vi "SubPanelAdd.vi"(0 "Add in":refnum<class "Add.lvclass">, 1 "B":dbl, 5 "A":dbl, 7 "user event out":refnum<user-event>, 9 "event source":refnum<user-event>, 11 "error in (no error)":errorcluster, 12 "Calculate":bool) -> (4 "Add out":refnum<class "Add.lvclass">, 6 "C":dbl, 15 "error out":errorcluster)   [LabVIEW 2023, in "Add.lvclass"]
uses:
  Add.lvclass
  Arithmetic/Arithmetic.lvclass
  Add.lvclass/Add.ctl
panel:
  # "ADDITION"
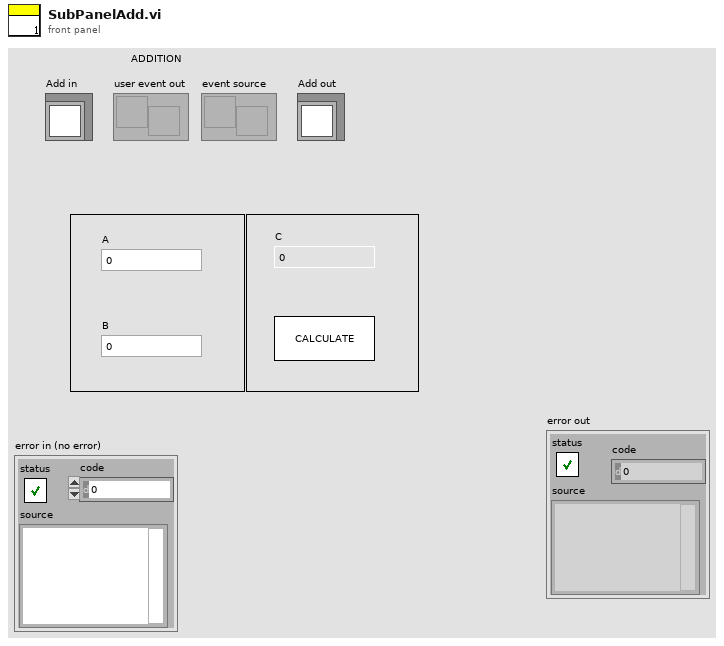
[diagram p1: front panel]
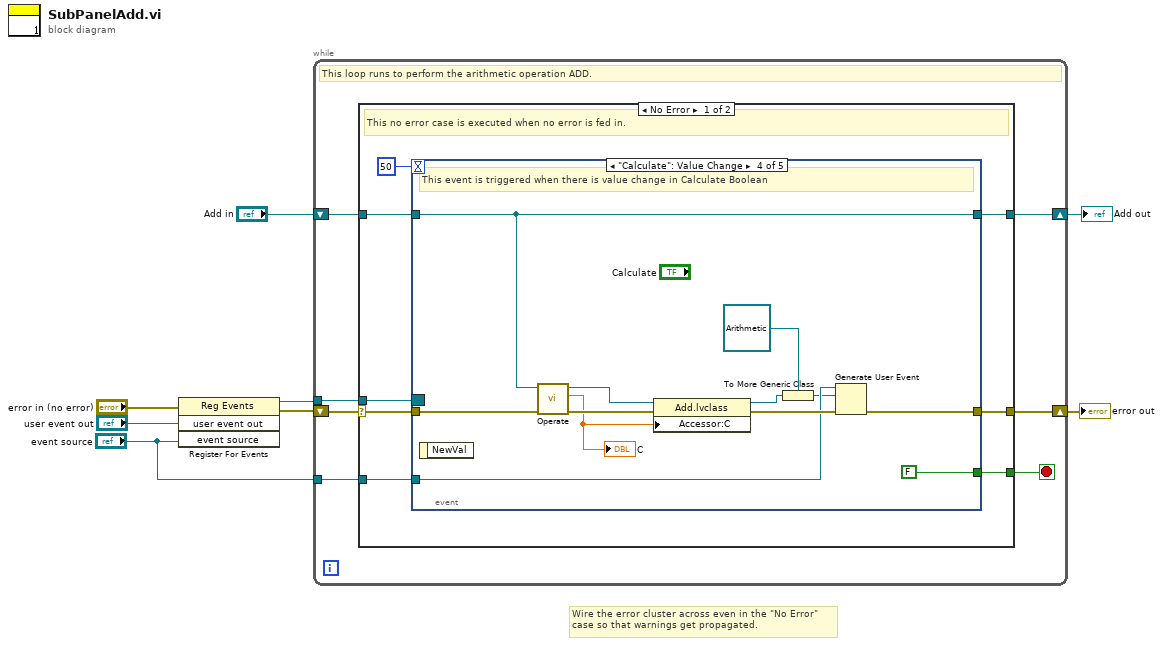
[diagram p0: block diagram]
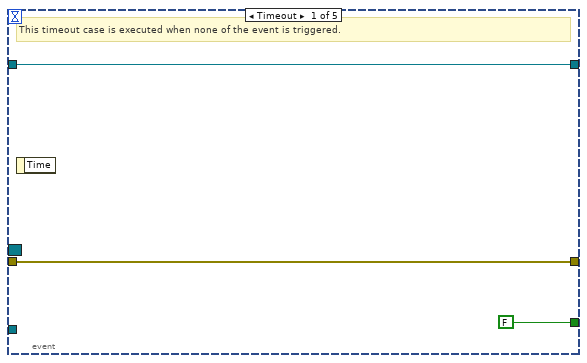
[diagram p2: hidden frame]
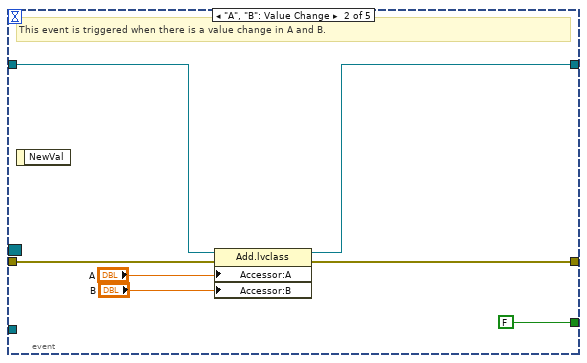
[diagram p3: hidden frame]
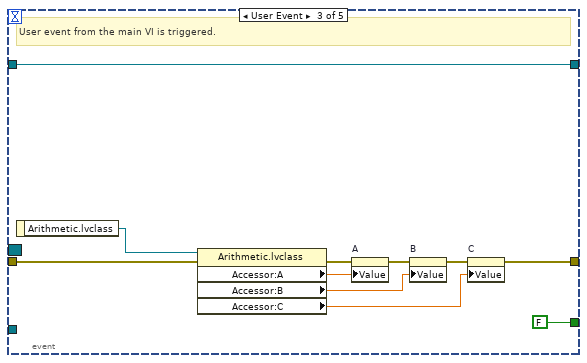
[diagram p4: hidden frame]
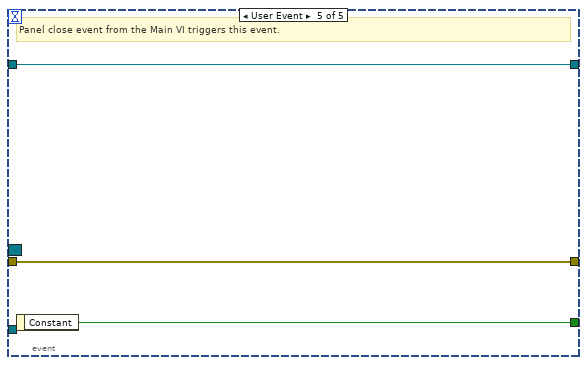
[diagram p5: hidden frame]
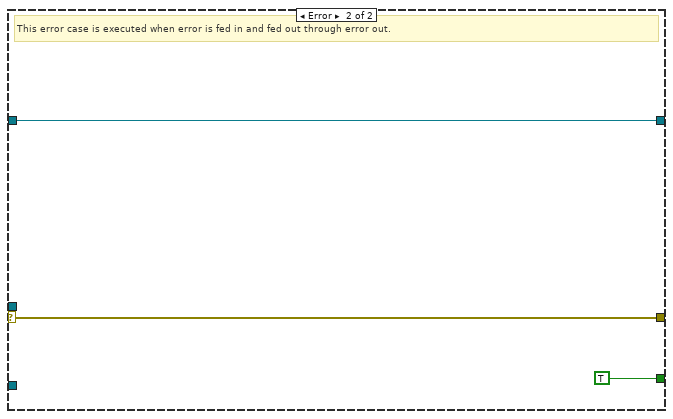
[diagram p6: hidden frame]
diagram:
  # "Wire the error cluster across even in the \"No Error\"\ncase so that warnings get propagated."
  n1 = register-events(error in="error in (no error)", "user event out", "event source") -> (reference out=w1:refnum<event-registration>, error out=w6:errorcluster)  [unwired: 1 in]
  n2 = while {
    shift-right: [w14] -> w4
    shift-left: w6 -> [w15]
    shift-right: [w12] -> w7
    shift-left: "Add in" -> [w13]
    tunnel: w1 -> [w11]
    tunnel: "event source" -> [w9]
    stop <- w10 stop-if-true
    # "This loop runs to perform the arithmetic operation ADD."
    n3 = case shown="No Error" w15 {
      selector: w15 -> [w23 w62]
      tunnel: [w22 w62] -> w14
      tunnel: [w20 w61] -> w12
      tunnel: w13 -> [w21 w61]
      tunnel: w11 -> [w18 _]
      tunnel: [w17 TRUE] -> w10
      tunnel: w9 -> [w16 _]
      frame No Error {
        # "This no error case is executed when no error is fed in."
        n4 = event shown="[3] \"Calculate\": Value Change" {
          selector: w18 -> [_ _ _ _ _]
          dyn-events: _ -> [_ _ _ _ _]
          timeout: 50 -> [_ _ _ _ _]
          tunnel: w23 -> [w26 w33 w44 w56 w59]
          tunnel: [w26 w32 w43 w53 w59] -> w22
          tunnel: w21 -> [w25 w28 w41 w47 w58]
          tunnel: [w25 w27 w41 w47 w58] -> w20
          tunnel: [FALSE FALSE FALSE ("Constant") FALSE w57] -> w17
          tunnel: w16 -> [_ _ _ w48 _]
          event Timeout {
            # "This timeout case is executed when none of the event is triggered."
            n5 = event-data() -> ()  [unwired: 1 in, 1 out]
          }
          event "A", "B": Value Change {
            # "This event is triggered when there is a value change in A and B."
            n6 = event-data() -> ()  [unwired: 1 in, 1 out]
            n7 = property class="Add.lvclass"(reference=w28, error in=w33, "Accessor:A"="A", "Accessor:B"="B") -> (reference out=w27:refnum<class "Add.lvclass">, error out=w32:errorcluster)
          }
          event User Event {
            # "User event from the main VI is triggered."
            n8 = event-data() -> ("Arithmetic.lvclass"=w34:refnum<class "Arithmetic.lvclass">)  [unwired: 1 in]
            n9 = property class="Arithmetic.lvclass"(reference=w34, error in=w44) -> (error out=w40:errorcluster, "Accessor:A"=w39:dbl, "Accessor:B"=w36:dbl, "Accessor:C"=w35:dbl)  [unwired: 1 out]
            n10 = property on="A" class="DigNum (strict)"(error in=w40, "Value"=w39) -> (error out=w38:errorcluster)  [unwired: 1 in, 1 out]
            n11 = property on="B" class="DigNum (strict)"(error in=w38, "Value"=w36) -> (error out=w37:errorcluster)  [unwired: 1 in, 1 out]
            n12 = property on="C" class="DigNum (strict)"(error in=w37, "Value"=w35) -> (error out=w43:errorcluster)  [unwired: 1 in, 1 out]
          }
          event "Calculate": Value Change {
            # "This event is triggered when there is value change in Calculate Boolean"
            n13 = event-data() -> ()  [unwired: 1 in, 1 out]
            n14 = call-dynamic "Operate.vi"("error in (no error)"=w56, "Add in"=w47) -> ("error out"=w54:errorcluster, "C"=w50:dbl, "Add out"=w51:refnum<class "Add.lvclass">)  [unwired: 7 in]
            "C" <- w50
            n15 = property class="Add.lvclass"(reference=w51, error in=w54, "Accessor:C"=w50) -> (reference out=w49:refnum<class "Add.lvclass">, error out=w52:errorcluster)
            n16 = To More Generic Class(target class=refnum<class "Arithmetic.lvclass"> refnum ("Arithmetic.lvclass"), reference=w49) -> (generic class reference=w46:refnum<class "Arithmetic.lvclass">)
            n17 = Generate User Event(user event=w48, event data cluster=w46, error in=w52) -> (error out=w53:errorcluster)  [unwired: 1 in, 1 out]
          }
          event User Event {
            # "Panel close event from the Main VI triggers this event."
            n18 = event-data() -> ("Constant"=w57:bool)  [unwired: 1 in]
          }
        }
      }
      frame Error {
        # "This error case is executed when error is fed in and fed out through error out."
      }
    }
  }
  "error out" <- w4
  "Add out" <- w7
